vi "ELait03.vi"(4 "error in":T13, 7 "Command":T14) -> (0 "error out":T13, 3 "Response":T11)   [LabVIEW 2018]
uses:
  MOKO_LabViewLibrary/MokoLowLevel/MokoLowLovelControl/MLLC_Command.ctl
  MOKO_LabViewLibrary/MokoLowLevel/MokoLowLovelControl/MLLC_Error.ctl
  MOKO_LabViewLibrary/MokoLowLevel/MokoLowLovelControl/MLLC_Mode.ctl
  MOKO_LabViewLibrary/MokoLowLevel/MokoLowLovelControl/MLLC_Response.ctl
  MOKO_LabViewLibrary/MokoLowLevel/MokoLowLovelControl/MLLC_DriverName.ctl
  MOKO_LabViewLibrary/MokoLowLevel/MokoLowLovelControl/MLLC_ResponseInit.ctl
  MOKO_LabViewLibrary/MokoLowLevel/MokoLowLovelControl/MLLC_Request.ctl
  MOKO_LabViewLibrary/MokoLowLevel/MokoLowLovelControl/MLLC_ErrorCode.ctl
  MOKO_LabViewLibrary/MokoLowLevel/MokoLowLovelControl/MLLC_ConnectCluster.ctl
  MOKO_LabViewLibrary/MokoLowLevel/MokoLowLovelControl/MLLC_InterfaceType.ctl
  MOKO_LabViewLibrary/MokoLowLevel/MokoLowLovelControl/MLLC_OpenedSession.ctl
  MOKO_LabViewLibrary/MokoLowLevel/MokoLowLovelControl/MLLC_InterfaceSettings.ctl
  MOKO_LabViewLibrary/MokoLowLevel/MokoLowLovelControl/MLLC_InterfaceKind.ctl
  MOKO_LabViewLibrary/MokoLowLevel/MokoLowLovelControl/MLLC_Rs232Settings.ctl
panel:
  in  "Settings":T6={"Permanent data"={"Connect"={"InterfaceType"=enum."VISA", "OpenedSession"="COM4", "InterfaceSettings"={"Interface"=enum."RS232", "EOS 4 read"=enum."Default (=EOS 4 write)", "EOS 4 write"=enum."CR (\\r)", "TMO, ms"=500, "Sett"=variant(cluster{"Baud Rate":u32, "Data Bits":u16, "Parity":u16, "Stop Bits":u16, "Flow Control":u16, "Eho":bool} {"Baud Rate"=75, "Data Bits"=0, "Parity"=0, "Stop Bits"=0, "Flow Control"=0, "Eho"=FALSE})}}, "Array - Value"=[], "Array - Time"=[], "Value critical"=0.0}, "Saved Data"=variant} {"Permanent data"."Value critical" format="%#_6f"}
  in  "Error Code":T7=5420
  in  "Request":T8="?MOD"
  in  "ResponseInit":T9="XP2I"
  in  "Driver Name":T10="Elait03"
  in  "Mode":T12=enum."Check"
  # "Elait03"
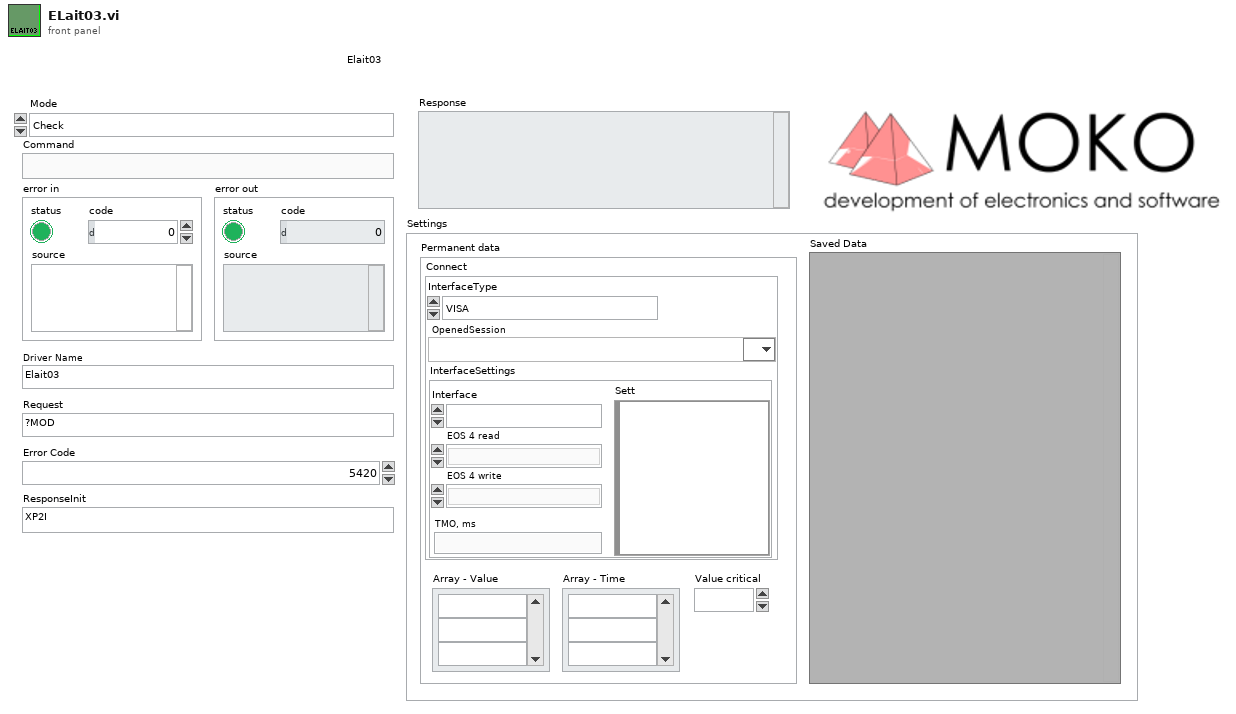
[diagram p1: front panel]
types:
  T1 = typedef "MLLC_ConnectCluster.ctl" = cluster{"InterfaceType":T2, "OpenedSession":T3, "InterfaceSettings":T4}
  T2 = typedef "MLLC_InterfaceType.ctl" = enum16{"VISA", "Prologix USB-GPIB"}
  T3 = typedef "MLLC_OpenedSession.ctl" = refnum<visa-resource-name>
  T4 = typedef "MLLC_InterfaceSettings.ctl" = cluster{"Interface":T5, "EOS 4 read":enum16{"Default (=EOS 4 write)", "CR (\\r)", "LF (\\n)", "None"}, "EOS 4 write":enum16{"CR+LF (\\r\\n)", "CR (\\r)", "LF (\\n)", "None"}, "TMO, ms":i32, "Sett":variant}
  T5 = typedef "MLLC_InterfaceKind.ctl" = enum16{"RS232", "GPIB", "USB", "Ethernet", "another"}
  T6 = cluster{"Permanent data":cluster{"Connect":T1, "Array - Value":string[], "Array - Time":string[], "Value critical":sgl}, "Saved Data":variant}
  T7 = typedef "MLLC_ErrorCode.ctl" = u32
  T8 = typedef "MLLC_Request.ctl" = string
  T9 = typedef "MLLC_ResponseInit.ctl" = string
  T10 = typedef "MLLC_DriverName.ctl" = string
  T11 = typedef "MLLC_Response.ctl" = string
  T12 = typedef "MLLC_Mode.ctl" = enum16{"get", "set", "close", "Init", "Check"}
  T13 = typedef "MLLC_Error.ctl" = errorcluster
  T14 = typedef "MLLC_Command.ctl" = string
  T15 = cluster{"Connect":T1, "Array - Value":string[], "Array - Time":string[], "Value critical":sgl}
  T16 = typedef "MLLC_Rs232Settings.ctl" = cluster{"Baud Rate":u32, "Data Bits":u16, "Parity":u16, "Stop Bits":u16, "Flow Control":u16, "Eho":bool, "Address":dbl}
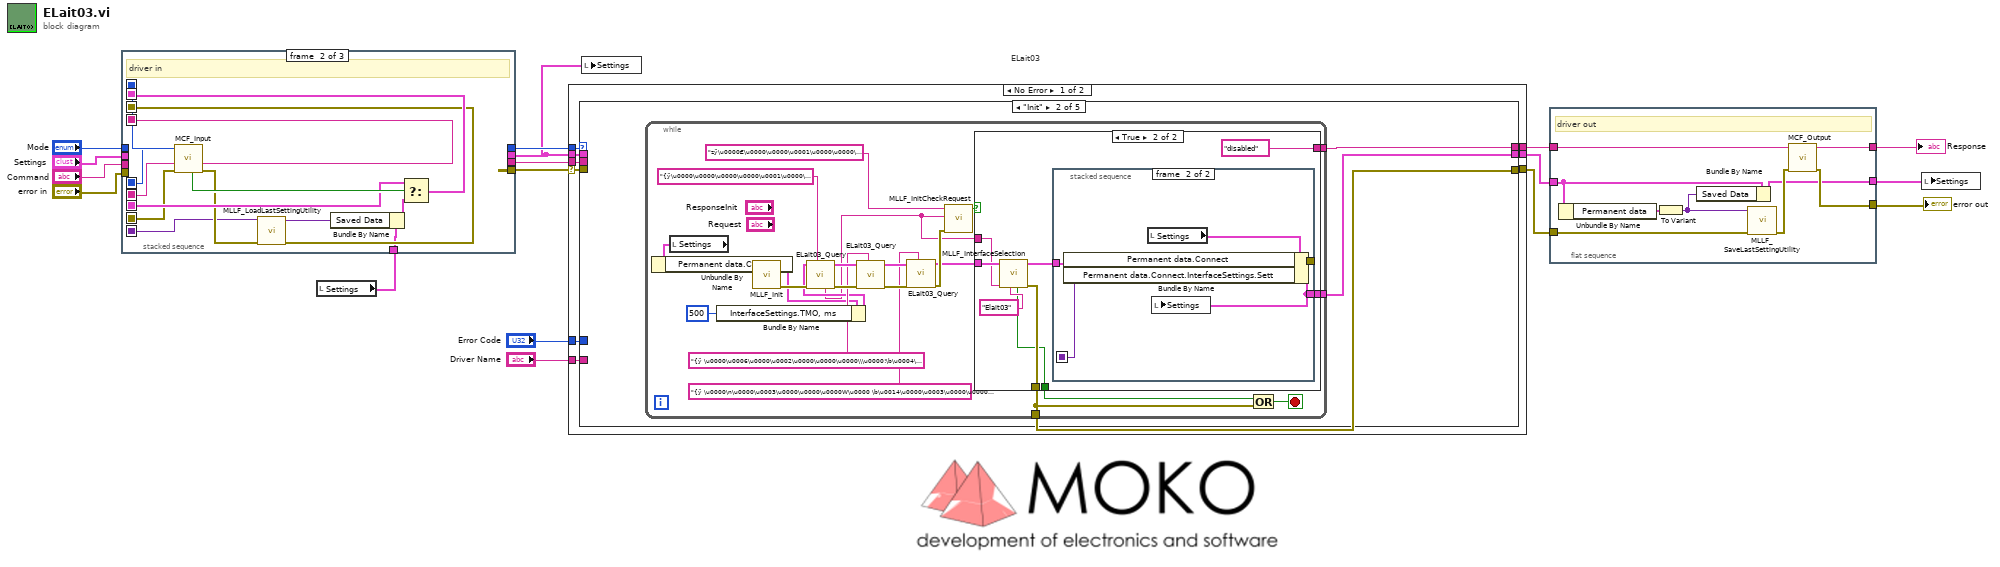
[diagram p0: block diagram]
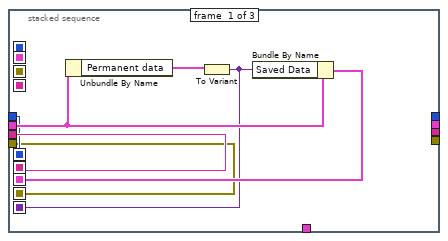
[diagram p2: hidden frame]
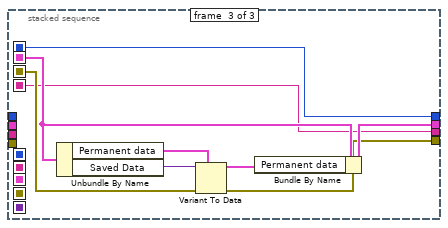
[diagram p3: hidden frame]
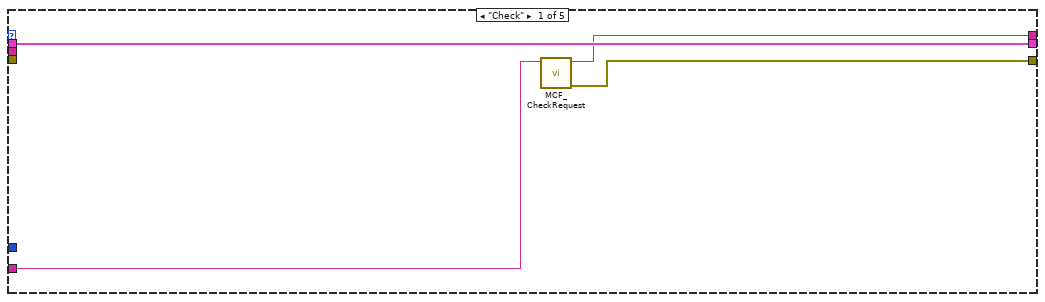
[diagram p4: hidden frame]
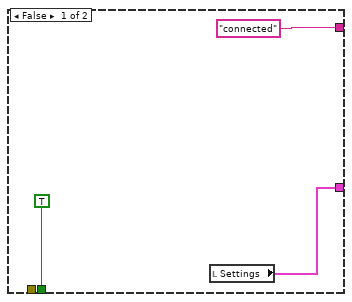
[diagram p5: hidden frame]
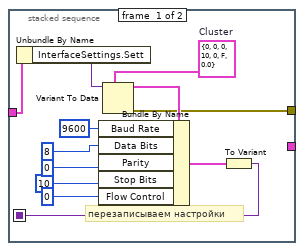
[diagram p6: hidden frame]
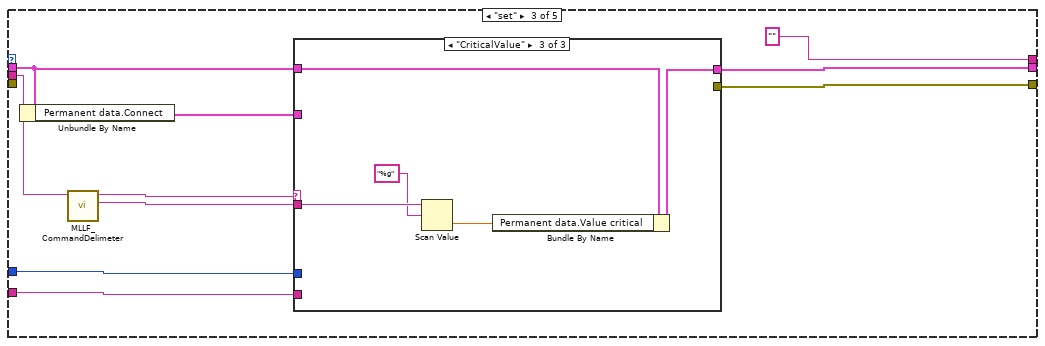
[diagram p7: hidden frame]
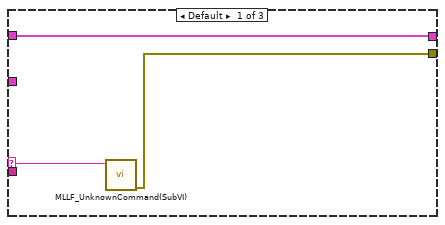
[diagram p8: hidden frame]
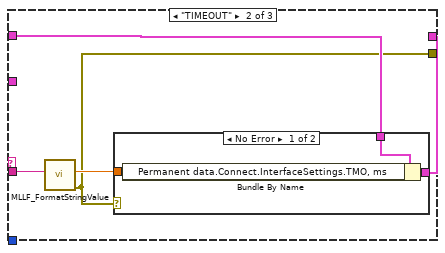
[diagram p9: hidden frame]
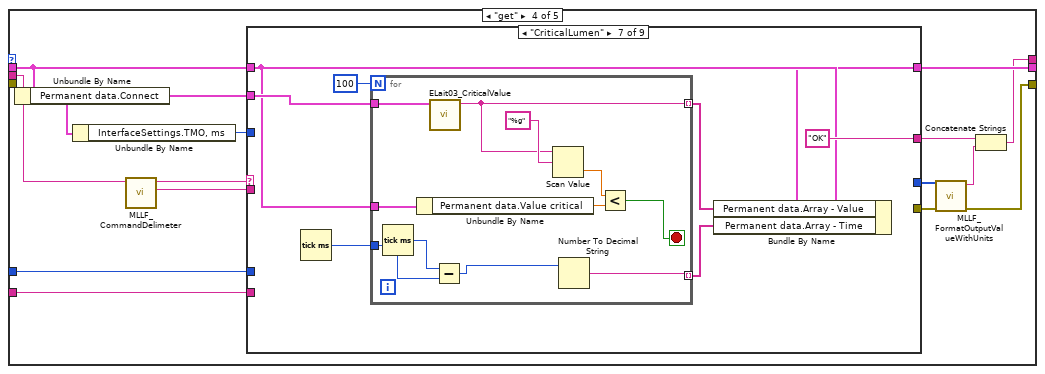
[diagram p11: hidden frame]
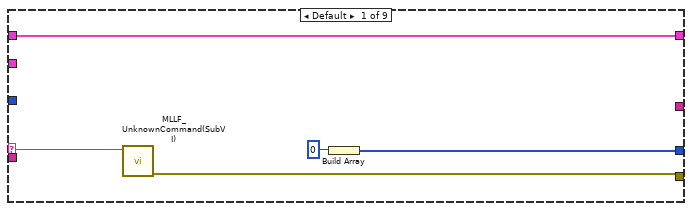
[diagram p12: hidden frame]
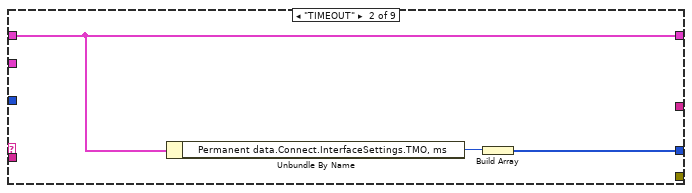
[diagram p13: hidden frame]
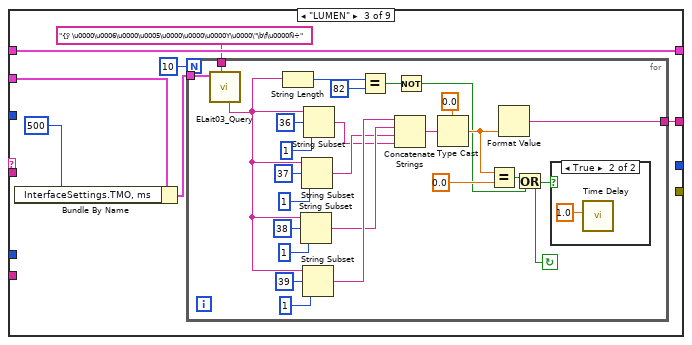
[diagram p14: hidden frame]
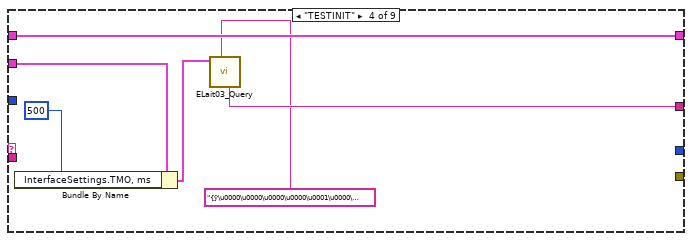
[diagram p16: hidden frame]
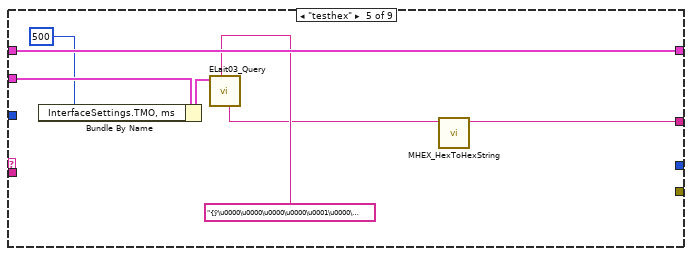
[diagram p17: hidden frame]
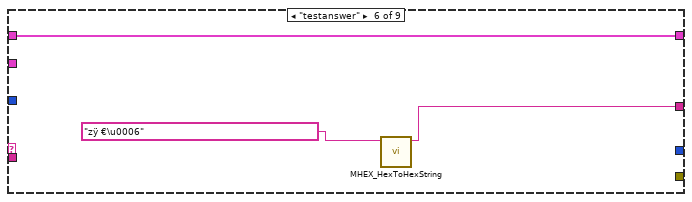
[diagram p18: hidden frame]
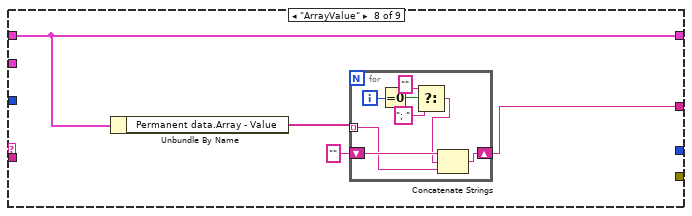
[diagram p19: hidden frame]
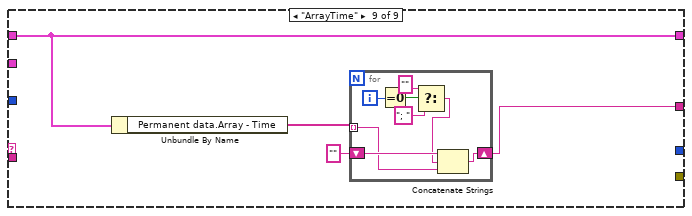
[diagram p20: hidden frame]
diagram:
  # "ELait03"
  n1 = local read "Settings"() -> (w11:T6)
  n2 = stacked-sequence {
    seq-local: [w20 _ _] -> [_ w36 _]
    seq-local: [w19 _ _] -> [_ w37 _]
    seq-local: [w22 _ _] -> [_ w32 _]
    seq-local: [w18 _ _] -> [_ w31 _]
    seq-local: [w21 _ _] -> [_ w27 _]
    seq-local: [_ w28 _] -> [_ _ w44]
    seq-local: [_ w38 _] -> [_ _ w41]
    seq-local: [_ w35 _] -> [_ _ w40]
    seq-local: [_ w34 _] -> [_ _ w45]
    tunnel: "Command" -> [w20 _ _]
    tunnel: "Mode" -> [w19 _ _]
    tunnel: "error in" -> [w18 _ _]
    tunnel: "Settings" -> [w23 _ _]
    tunnel: w11 -> [_ w26 _]
    tunnel: [_ _ w40] -> w8
    tunnel: [_ _ w43] -> w9
    tunnel: [_ _ w42] -> w7
    tunnel: [_ _ w41] -> w10
    frame #0 {
      n3 = Unbundle By Name(w23) -> ("Permanent data"=w24:T15)
      n4 = To Variant(anything=w24) -> (Variant=w21:variant)
      n5 = Bundle By Name(cluster=w23, "Saved Data"=w21) -> (w22:T6)
    }
    frame #1 {
      # "driver in"
      n6 = call "MCF_Input.vi"("Error In"=w31, "Command in"=w36, "Mode in"=w37) -> ("Error Out"=w30:errorcluster, "Command out"=w35:string, "Mode out"=w38:T12, "Boolean"=w33:bool)  [unwired: 5 in]
      n7 = call "MLLF_LoadLastSettingUtility.vi"("Error In"=w30, "Save data in"=w27) -> ("Error Out"=w28:errorcluster, "Save data out"=w25:variant)  [unwired: 8 in]
      n8 = Bundle By Name(cluster=w26, "Saved Data"=w25) -> (w29:T6)
      n9 = Select(t=w32, s=w33, f=w29) -> (s? t:f=w34:T6)
    }
    frame #2 {
      n10 = Unbundle By Name(w45) -> ("Permanent data"=w46:T15, "Saved Data"=w39:variant)
      n11 = Variant To Data(error in=w44, type=w46, Variant=w39) -> (data=w47:T15, error out=w42:errorcluster)
      n12 = Bundle By Name(cluster=w45, "Permanent data"=w47) -> (w43:T6)
    }
  }
  n13 = case shown="No Error" w7 {
    selector: w7 -> [w53 w262]
    tunnel: [w48 w262] -> w4
    tunnel: w10 -> [w56 _]
    tunnel: [w55 _] -> w6
    tunnel: w8 -> [w54 _]
    tunnel: w9 -> [w50 w261]
    tunnel: "Error Code" -> [w52 _]
    tunnel: "Driver Name" -> [w51 _]
    tunnel: [w49 w261] -> w5
    frame No Error {
      n14 = case shown="\"Init\"" w56 {
        tunnel: [w58 w63 "" ("Output String") w142 "" ("Output String")] -> w55
        tunnel: w54 -> [_ _ w117 w146 _]
        tunnel: w53 -> [_ _ _ _ _]
        tunnel: w52 -> [_ _ w123 w154 _]
        tunnel: w51 -> [w59 _ w120 w153 _]
        tunnel: w50 -> [w60 _ w122 w155 w259]
        tunnel: [w60 w62 w121 w152 w259] -> w49
        tunnel: [w57 w61 w114 w141 w258] -> w48
        frame "Check" {
          n15 = call "MCF_CheckRequest.vi"("Driver Name"=w59) -> ("Error Out"=w57:errorcluster, "Output String"=w58:string)  [unwired: 9 in]
        }
        frame "Init" {
          n16 = while {
            tunnel: [w83] -> w61
            tunnel: [w82] -> w63
            tunnel: [w81] -> w62
            stop <- w85 stop-if-true
            n17 = local read "Settings"() -> (w79:T6)
            n18 = Unbundle By Name(w79) -> ("Permanent data.Connect"=w78:T1)
            n19 = call "MLLF_Init.vi"("DriverConnect in"=w78) -> ("Error Out"=w86:errorcluster, "DriverConnect out"=w67:T1)  [unwired: 7 in]
            n20 = Bundle By Name(cluster=w67, "InterfaceSettings.TMO, ms"=500) -> (w66:T1)
            n21 = call "ELait03_Query.vi"("String"="{ÿ\u0000\u0000\u0000\u0000\u0001\u0000\u0000\u0000ƒ\u0000", "error in (no error)"=w86, "DriverConnect in"=w66) -> ("error out"=w75:errorcluster, "DriverConnect out"=w74:T1, "String from device out"=w64:string)  [unwired: 6 in]
            n22 = call "ELait03_Query.vi"("String"="{ÿ \u0000\u0006\u0000\u0002\u0000\u0000\u0000\\\u0000!\b\u0004\u0000Ú÷", "error in (no error)"=w75, "DriverConnect in"=w74) -> ("error out"=w72:errorcluster, "DriverConnect out"=w73:T1)  [unwired: 6 in, 1 out]
            n23 = call "ELait03_Query.vi"("String"="{ÿ \u0000\n\u0000\u0003\u0000\u0000\u0000W\u0000 \b\u0014\u0000\u0003\u0000\u0000\u0000È÷", "error in (no error)"=w72, "DriverConnect in"=w73) -> ("error out"=w71:errorcluster, "DriverConnect out"=w68:T1)  [unwired: 6 in, 1 out]
            n24 = call "MLLF_InitCheckRequest.vi"("error in (no error)"=w71, "Answer"=w64, "Response Init"="zÿ\u0000€\u0000\u0000\u0001\u0000\u0000\u0000ƒ€") -> ("Design"=w80:bool)  [unwired: 5 in, 3 out]
            n25 = case shown="True" w80 {
              tunnel: w68 -> [_ w96]
              tunnel: [TRUE w92] -> w84
              tunnel: [_ w97] -> w83
              tunnel: ["connected" "disabled"] -> w82
              tunnel: [w87 w91] -> w81
              tunnel: w64 -> [_ w90]
              frame False {
                n26 = local read "Settings"() -> (w87:T6)
              }
              frame True {
                n27 = call "MLLF_InterfaceSelection.vi"("Driver Name"="Elait03" ("String"), "Answer:"=w90, "DriverConnect in"=w96) -> ("error out"=w97:T13, "DriverConnect out"=w95:T1, "stop init?"=w92:bool)  [unwired: 4 in, 2 out]
                n28 = stacked-sequence {
                  seq-local: [w101 _] -> [_ w110]
                  tunnel: w95 -> [w99 w111]
                  tunnel: [w102 _] -> _
                  tunnel: [_ w112] -> w91
                  frame #0 {
                    w103 = T16 {"Baud Rate"=0, "Data Bits"=0, "Parity"=0, "Stop Bits"=10, "Flow Control"=0, "Eho"=FALSE, "Address"=0.0}  # Cluster
                    # "перезаписываем настройки"
                    n29 = Unbundle By Name(w99) -> ("InterfaceSettings.Sett"=w98:variant)
                    n30 = Variant To Data(type=w103, Variant=w98) -> (data=w104:T16, error out=w102:errorcluster)  [unwired: 1 in]
                    n31 = Bundle By Name(cluster=w104, "Baud Rate"=u32 9600, "Data Bits"=u16 8 ("Serial Settings:Data Bits"), "Parity"=u16 0 ("Serial Settings:Parity"), "Stop Bits"=u16 10 ("Serial Settings:Stop Bits"), "Flow Control"=u16 0 ("Serial Settings:Flow Control")) -> (w109:T16)
                    n32 = To Variant(anything=w109) -> (Variant=w101:variant)
                  }
                  frame #1 {
                    n33 = local read "Settings"() -> (w113:T6)
                    n34 = Bundle By Name(cluster=w113, "Permanent data.Connect"=w111, "Permanent data.Connect.InterfaceSettings.Sett"=w110) -> (w112:T6)
                    n35 = local write "Settings"(w112) -> ()
                  }
                }
              }
            }
            n36 = Or(x=w84, y=w83) -> (x .or. y?=w85:bool)
          }
        }
        frame "set" {
          n37 = Unbundle By Name(w122) -> ("Permanent data.Connect"=w118:T1)
          n38 = call "MLLF_CommandDelimeter.vi"("command with param"=w117) -> ("param 1"=w115:string, "command"=w116:string)  [unwired: 6 in, 3 out]
          n39 = case shown="\"CriticalValue\"" w116 {
            selector: w116 -> [w125 _ _]
            tunnel: w115 -> [_ w129 w138]
            tunnel: w123 -> [_ _ _]
            tunnel: w122 -> [w126 w130 w140]
            tunnel: [w126 w131 w139] -> w121
            tunnel: w120 -> [_ _ _]
            tunnel: [w124 w127 _] -> w114
            tunnel: w118 -> [_ _ _]
            frame Default {
              n40 = call "MLLF_UnknownCommand(SubVI).vi"("Unknown command"=w125) -> ("error out"=w124:errorcluster)  [unwired: 10 in]
            }
            frame "TIMEOUT" {
              n41 = call "MLLF_FormatStringValue.vi"("String Value"=w129) -> ("error out"=w127:T13, "number"=w128:dbl)  [unwired: 8 in, 1 out]
              n42 = case shown="No Error" w127 {
                tunnel: [w134 w135] -> w131
                tunnel: w130 -> [w133 w135]
                tunnel: w128 -> [w132 _]
                frame No Error {
                  n43 = Bundle By Name(cluster=w133, "Permanent data.Connect.InterfaceSettings.TMO, ms"=w132) -> (w134:T6)
                }
                frame Error {
                }
              }
            }
            frame "CriticalValue" {
              n44 = Scan Value(string=w138, format string="%g") -> (value=w137:dbl)  [unwired: 1 in, 1 out]
              n45 = Bundle By Name(cluster=w140, "Permanent data.Value critical"=w137) -> (w139:T6)
            }
          }
        }
        frame "get" {
          n46 = Unbundle By Name(w155) -> ("Permanent data.Connect"=w143:T1)
          n47 = Unbundle By Name(w143) -> ("InterfaceSettings.TMO, ms"=w149:i32)
          n48 = call "MLLF_CommandDelimeter.vi"("command with param"=w146) -> ("param 1"=w144:string, "command"=w145:string)  [unwired: 6 in, 3 out]
          n49 = case shown="\"CriticalLumen\"" w145 {
            selector: w145 -> [w157 _ _ _ _ _ _ _ _]
            tunnel: w144 -> [_ _ _ _ _ _ _ _ _]
            tunnel: [w156 _ _ _ _ _ _ _ _] -> w151
            tunnel: w154 -> [_ _ _ _ _ _ _ _ _]
            tunnel: [w160 w163 w170 w203 w210 w211 w214 w234 w246] -> w152
            tunnel: w155 -> [w160 w163 w170 w203 w210 w211 w217 w234 w246]
            tunnel: [w158 w161 _ _ _ _ _ _ _] -> w150
            tunnel: w153 -> [_ _ _ _ _ _ _ _ _]
            tunnel: w149 -> [_ _ _ _ _ _ _ _ _]
            tunnel: [_ _ w168 w199 w204 w212 "OK" ("output string") w233 w245] -> w147
            tunnel: w143 -> [_ _ w166 w202 w209 _ w221 _ _]
            frame Default {
              n50 = call "MLLF_UnknownCommand(SubVI).vi"("Unknown command"=w157) -> ("error out"=w156:errorcluster)  [unwired: 10 in]
              n51 = Build Array(0 ("TimeOut")) -> (w158:i32[])
            }
            frame "TIMEOUT" {
              n52 = Unbundle By Name(w163) -> ("Permanent data.Connect.InterfaceSettings.TMO, ms"=w162:i32)
              n53 = Build Array(w162) -> (w161:i32[])
            }
            frame "LUMEN" {
              n54 = Bundle By Name(cluster=w166, "InterfaceSettings.TMO, ms"=500) -> (w164:T1)
              n55 = for {
                N: 10 -> [_]
                tunnel: w164 -> [w182]
                tunnel: "{ÿ \u0000\u0006\u0000\u0005\u0000\u0000\u0000Y\u0000\"\b\f\u0000Ñ÷" -> [w181]
                tunnel: [w180] -> w168
                stop <- w171 continue-if-true
                n56 = call "ELait03_Query.vi"("String"=w181, "DriverConnect in"=w182) -> ("String from device out"=w179:string)  [unwired: 7 in, 2 out]
                n57 = String Length(string=w179) -> (length=w178:i32)
                n58 = String Subset(string=w179, offset (0)=38, length (rest)=1 ("length (rest)")) -> (substring=w186:string)
                n59 = String Subset(string=w179, offset (0)=37, length (rest)=1 ("length (rest)")) -> (substring=w185:string)
                n60 = String Subset(string=w179, offset (0)=39, length (rest)=1 ("length (rest)")) -> (substring=w187:string)
                n61 = String Subset(string=w179, offset (0)=36, length (rest)=1 ("length (rest)")) -> (substring=w184:string)
                n62 = Equal?(x=w178, y=82) -> (x = y?=w176:bool)
                n63 = Concatenate Strings(w187, w186, w185, w184) -> (w183:string)
                n64 = Not(x=w176) -> (.not. x?=w172:bool)
                n65 = Type Cast(type=sgl 0.0, x=w183) -> (*(type *) &x=w175:sgl)
                n66 = Equal?(x=w175, y=sgl 0.0) -> (x = y?=w173:bool)
                n67 = Format Value(value (0)=w175) -> (output string=w180:string)  [unwired: 2 in]
                n68 = Or(x=w173, y=w172) -> (x .or. y?=w171:bool)
                n69 = case shown="True" w171 {
                  frame False {
                  }
                  frame True {
                    n70 = call "Time Delay"("Delay Time (s)"=1.0) -> ()  [unwired: 10 in, 1 out]
                  }
                }
              }
            }
            frame "TESTINIT" {
              n71 = Bundle By Name(cluster=w202, "InterfaceSettings.TMO, ms"=500) -> (w200:T1)
              n72 = call "ELait03_Query.vi"("String"="{ÿ\u0000\u0000\u0000\u0000\u0001\u0000\u0000\u0000ƒ\u0000", "DriverConnect in"=w200) -> ("String from device out"=w199:string)  [unwired: 7 in, 2 out]
            }
            frame "testhex" {
              n73 = Bundle By Name(cluster=w209, "InterfaceSettings.TMO, ms"=500) -> (w207:T1)
              n74 = call "ELait03_Query.vi"("String"="{ÿ\u0000\u0000\u0000\u0000\u0001\u0000\u0000\u0000ƒ\u0000", "DriverConnect in"=w207) -> ("String from device out"=w205:string)  [unwired: 7 in, 2 out]
              n75 = call "MHEX_HexToHexString.vi"("STRING HEX"=w205) -> ("String out"=w204:string)  [unwired: 8 in, 2 out]
            }
            frame "testanswer" {
              n76 = call "MHEX_HexToHexString.vi"("STRING HEX"="zÿ €\u0006") -> ("String out"=w212:string)  [unwired: 8 in, 2 out]
            }
            frame "CriticalLumen" {
              n77 = Tick Count (ms)() -> (millisecond timer value=w219:u32)
              n78 = for {
                N: 100 -> [_]
                tunnel: w221 -> [w232]
                tunnel: [w229] -> w216 mode=indexing
                tunnel: w217 -> [w231]
                tunnel: w219 -> [w224]
                tunnel: [w222] -> w215 mode=indexing
                stop <- w226 stop-if-true
                n79 = Tick Count (ms)() -> (millisecond timer value=w225:u32)
                n80 = Unbundle By Name(w231) -> ("Permanent data.Value critical"=w227:sgl)
                n81 = call "ELait03_CriticalValue.vi"("DriverConnect"=w232) -> ("output string"=w229:string)  [unwired: 10 in]
                n82 = Subtract(x=w225, y=w224) -> (x-y=w223:u32)
                n83 = Scan Value(string=w229, format string="%g") -> (value=w228:dbl)  [unwired: 1 in, 1 out]
                n84 = Number To Decimal String(number=w223) -> (decimal integer string=w222:string)  [unwired: 1 in]
                n85 = Less?(x=w228, y=w227) -> (x < y?=w226:bool)
              }
              n86 = Bundle By Name(cluster=w217, "Permanent data.Array - Value"=w216, "Permanent data.Array - Time"=w215) -> (w214:T6)
            }
            frame "ArrayValue" {
              n87 = Unbundle By Name(w234) -> ("Permanent data.Array - Value"=w235:string[])
              n88 = for {
                tunnel: w235 -> [w237] mode=indexing
                shift-right: [w243] -> w233
                shift-left: "" -> [w244]
                i -> [w242]
                n89 = Equal To 0?(x=w242) -> (x = 0?=w241:bool)
                n90 = Select(t="" ("string"), s=w241, f="; " ("string")) -> (s? t:f=w238:string)
                n91 = Concatenate Strings(w244, w238, w237) -> (w243:string)
              }
            }
            frame "ArrayTime" {
              n92 = Unbundle By Name(w246) -> ("Permanent data.Array - Time"=w247:string[])
              n93 = for {
                tunnel: w247 -> [w249] mode=indexing
                shift-right: [w255] -> w245
                shift-left: "" -> [w256]
                i -> [w254]
                n94 = Equal To 0?(x=w254) -> (x = 0?=w253:bool)
                n95 = Select(t="" ("string"), s=w253, f="; " ("string")) -> (s? t:f=w250:string)
                n96 = Concatenate Strings(w256, w250, w249) -> (w255:string)
              }
            }
          }
          n97 = call "MLLF_FormatOutputValueWithUnits.vi"("error in"=w151, "ValuesIn"=w150) -> ("error out"=w141:T13, "Result string"=w148:T14)  [unwired: 8 in]
          n98 = Concatenate Strings(w147, w148) -> (w142:string)
        }
        frame "close" {
          n99 = Unbundle By Name(w259) -> ("Permanent data.Connect.OpenedSession"=w260:T3)
          n100 = VISA Close(VISA resource name=w260) -> (error out=w258:errorcluster)  [unwired: 1 in]
        }
      }
    }
    frame Error {
    }
  }
  n101 = local write "Settings"(w9) -> ()
  n102 = flat-sequence {
    tunnel: [w271] -> w3
    tunnel: [w270] -> w2
    tunnel: w6 -> [w269]
    tunnel: w4 -> [w268]
    tunnel: w5 -> [w264]
    tunnel: [w266] -> w1
    frame #0 {
      # "driver out"
      n103 = Unbundle By Name(w264) -> ("Permanent data"=w263:T15)
      n104 = To Variant(anything=w263) -> (Variant=w265:variant)
      n105 = Bundle By Name(cluster=w264, "Saved Data"=w265) -> (w266:T6)
      n106 = call "MLLF_SaveLastSettingUtility.vi"("error in"=w268, "Saved Data"=w265) -> ("error out"=w267:T13)  [unwired: 8 in, 1 out]
      n107 = call "MCF_Output.vi"("Error In"=w267, "Input"=w269) -> ("Error Out"=w270:errorcluster, "Output"=w271:string)  [unwired: 8 in]
    }
  }
  n108 = local write "Settings"(w1) -> ()
  "error out" <- w2
  "Response" <- w3
